vi "Timed relay switch.vi"() -> ()   [LabVIEW 2017]
uses:
  <vilib>/Platform/TimedLoop/XDataNode/timing_clust.ctl
  <vilib>/Platform/TimedLoop/XDataNode/nitl_modes.ctl
  <vilib>/Platform/TimedLoop/XDataNode/wakeup.ctl
  <vilib>/DAQmx/write.llb/DAQmx Write (Digital Bool 1Line 1Point).vi
  <vilib>/DAQmx/create/channels.llb/DAQmx Create Channel (DO-Digital Output).vi
  <vilib>/DAQmx/miscellaneous.llb/DAQmx Fill In Error Info.vi
  <vilib>/Platform/TimedLoop/XDataNode/XDataNode.xnode
  <vilib>/Platform/TimedLoop/XDataNode/XDNodeRunTimeDep.lvlib
panel:
  in  "stop":bool
  in  "On Time":i64=1000
  out "counter":i8
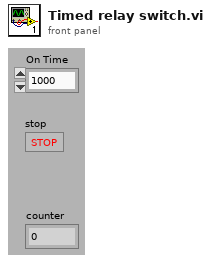
[diagram p1: front panel]
types:
  T1 = typedef "XDNodeRunTimeDep.lvlib/timing_clust.ctl" = cluster{"Expected End [f-1]":u64, "Actual End [f-1]":u64, "Finished Late? [f-1]":bool, "Expected End [i-1]":u64, "Actual End [i-1]":u64, "Finished Late? [i-1]":bool, "Expected Start [i]":u64, "Actual Start [i]":u64, "Expected Start [f]":u64, "Actual Start [f]":u64, "Source Name":string, "Structure Name":string, "Period":i64, "Deadline":i64, "Offset":i64, "Start":i64, "Priority":i32, "Timeout":i32, "Mode":T2, "Wakeup Reason":T3, "Error":errorcluster, "Source Type":string, "Secondary Source Type":string, "Global End Time":u64, "Global Start Time":u64, "Frame Duration":u64, "Iteration Duration":u64, "Assigned CPU":i32, "I/O Scan Engine Mode":u32}
  T2 = typedef "XDNodeRunTimeDep.lvlib/nitl_modes.ctl" = enum32{"No Change", "Process missed periods, maintain original phase", "Discard missed periods, maintain original phase", "Process missed periods, ignore original phase", "Discard missed periods, ignore original phase"}
  T3 = typedef "XDNodeRunTimeDep.lvlib/wakeup.ctl" = enum32{"Normal", "Aborted", "Asynchronous wakeup", "Timing source error", "Timed loop error", "Timeout"}
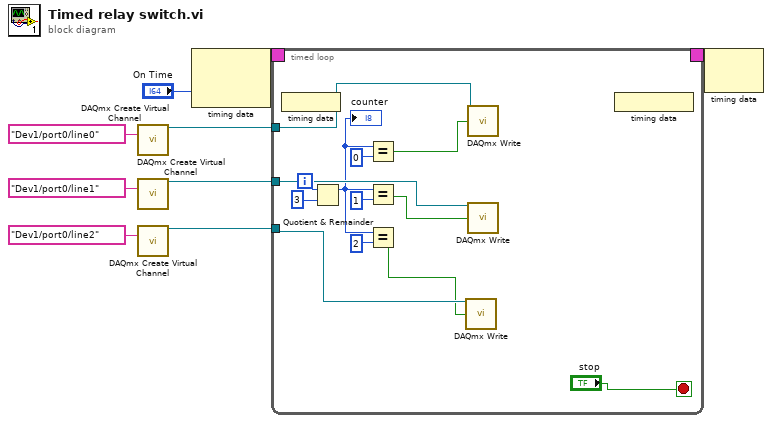
[diagram p0: block diagram]
diagram:
  n1 = call-poly <vilib>:"DAQmx Create Virtual Channel.vi"("lines"=tag "Dev1/port0/line0") -> ("task out"=w6:refnum<k21>)  [unwired: 5 in, 9 out]
  n2 = call-poly <vilib>:"DAQmx Create Virtual Channel.vi"("lines"=tag "Dev1/port0/line1") -> ("task out"=w5:refnum<k21>)  [unwired: 5 in, 9 out]
  n3 = call-poly <vilib>:"DAQmx Create Virtual Channel.vi"("lines"=tag "Dev1/port0/line2") -> ("task out"=w4:refnum<k21>)  [unwired: 5 in, 9 out]
  n4 = node-c288("On Time") -> (w3:T1)  [unwired: 1 out]
  n5 = timed-loop {
    timing: w3 -> [_]
    timing-out: [_] -> w2
    tunnel: w4 -> [w18]
    tunnel: w5 -> [w17]
    tunnel: w6 -> [w19]
    i -> [w21]
    stop <- "stop" stop-if-true
    n6 = node-c288() -> ()  [unwired: 1 out]
    n7 = Quotient & Remainder(x=w21, y=3) -> (x-y*floor(x/y)=w10:i32)  [unwired: 1 out]
    "counter" <- w10
    n8 = Equal?(x=w10, y=0) -> (x = y?=w16:bool)
    n9 = Equal?(x=w10, y=1) -> (x = y?=w15:bool)
    n10 = Equal?(x=w10, y=2) -> (x = y?=w14:bool)
    n11 = call-poly <vilib>:"DAQmx Write.vi"("task/channels in"=w18, "data"=w14) -> ()  [unwired: 2 in, 12 out]
    n12 = call-poly <vilib>:"DAQmx Write.vi"("task/channels in"=w19, "data"=w16) -> ()  [unwired: 2 in, 12 out]
    n13 = call-poly <vilib>:"DAQmx Write.vi"("task/channels in"=w17, "data"=w15) -> ()  [unwired: 2 in, 12 out]
    n14 = node-c288() -> ()  [unwired: 1 out]
  }
  n15 = node-c288(w2) -> ()  [unwired: 1 out]
